vi "Speed PI Control.vi"() -> ()   [LabVIEW 2016]
uses:
  <vilib>/Platform/TimedLoop/XDataNode/timing_clust.ctl
  <vilib>/Platform/TimedLoop/XDataNode/nitl_modes.ctl
  <vilib>/Platform/TimedLoop/XDataNode/wakeup.ctl
  <vilib>/platform/TimedLoop/XDataNode/XDataNode.xnode
  <vilib>/Platform/TimedLoop/XDataNode/XDNodeRunTimeDep.lvlib
panel:
  in  "I-Gain":dbl(slide)=1.0 scale=0.0..2.0
  in  "P-Gain":dbl(slide)=1.0 scale=0.0..2.0
  in  "Setpoint Speed (rps)":dbl(slide) scale=-8.3..8.3
  out "Speed (rps)":dynamicdata(graph)
  in  "stop (F)":bool
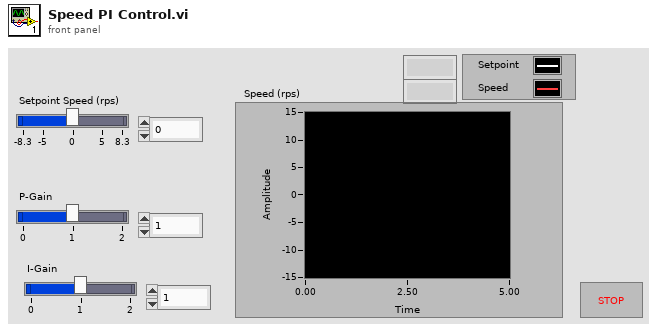
[diagram p1: front panel]
types:
  T1 = typedef "XDNodeRunTimeDep.lvlib/timing_clust.ctl" = cluster{"Expected End [f-1]":u64, "Actual End [f-1]":u64, "Finished Late? [f-1]":bool, "Expected End [i-1]":u64, "Actual End [i-1]":u64, "Finished Late? [i-1]":bool, "Expected Start [i]":u64, "Actual Start [i]":u64, "Expected Start [f]":u64, "Actual Start [f]":u64, "Source Name":string, "Structure Name":string, "Period":i64, "Deadline":i64, "Offset":i64, "Start":i64, "Priority":i32, "Timeout":i32, "Mode":T2, "Wakeup Reason":T3, "Error":errorcluster, "Source Type":string, "Secondary Source Type":string, "Global End Time":u64, "Global Start Time":u64, "Frame Duration":u64, "Iteration Duration":u64, "Assigned CPU":i32, "I/O Scan Engine Mode":u32}
  T2 = typedef "XDNodeRunTimeDep.lvlib/nitl_modes.ctl" = enum32{"No Change", "Process missed periods, maintain original phase", "Discard missed periods, maintain original phase", "Process missed periods, ignore original phase", "Discard missed periods, ignore original phase"}
  T3 = typedef "XDNodeRunTimeDep.lvlib/wakeup.ctl" = enum32{"Normal", "Aborted", "Asynchronous wakeup", "Timing source error", "Timed loop error", "Timeout"}
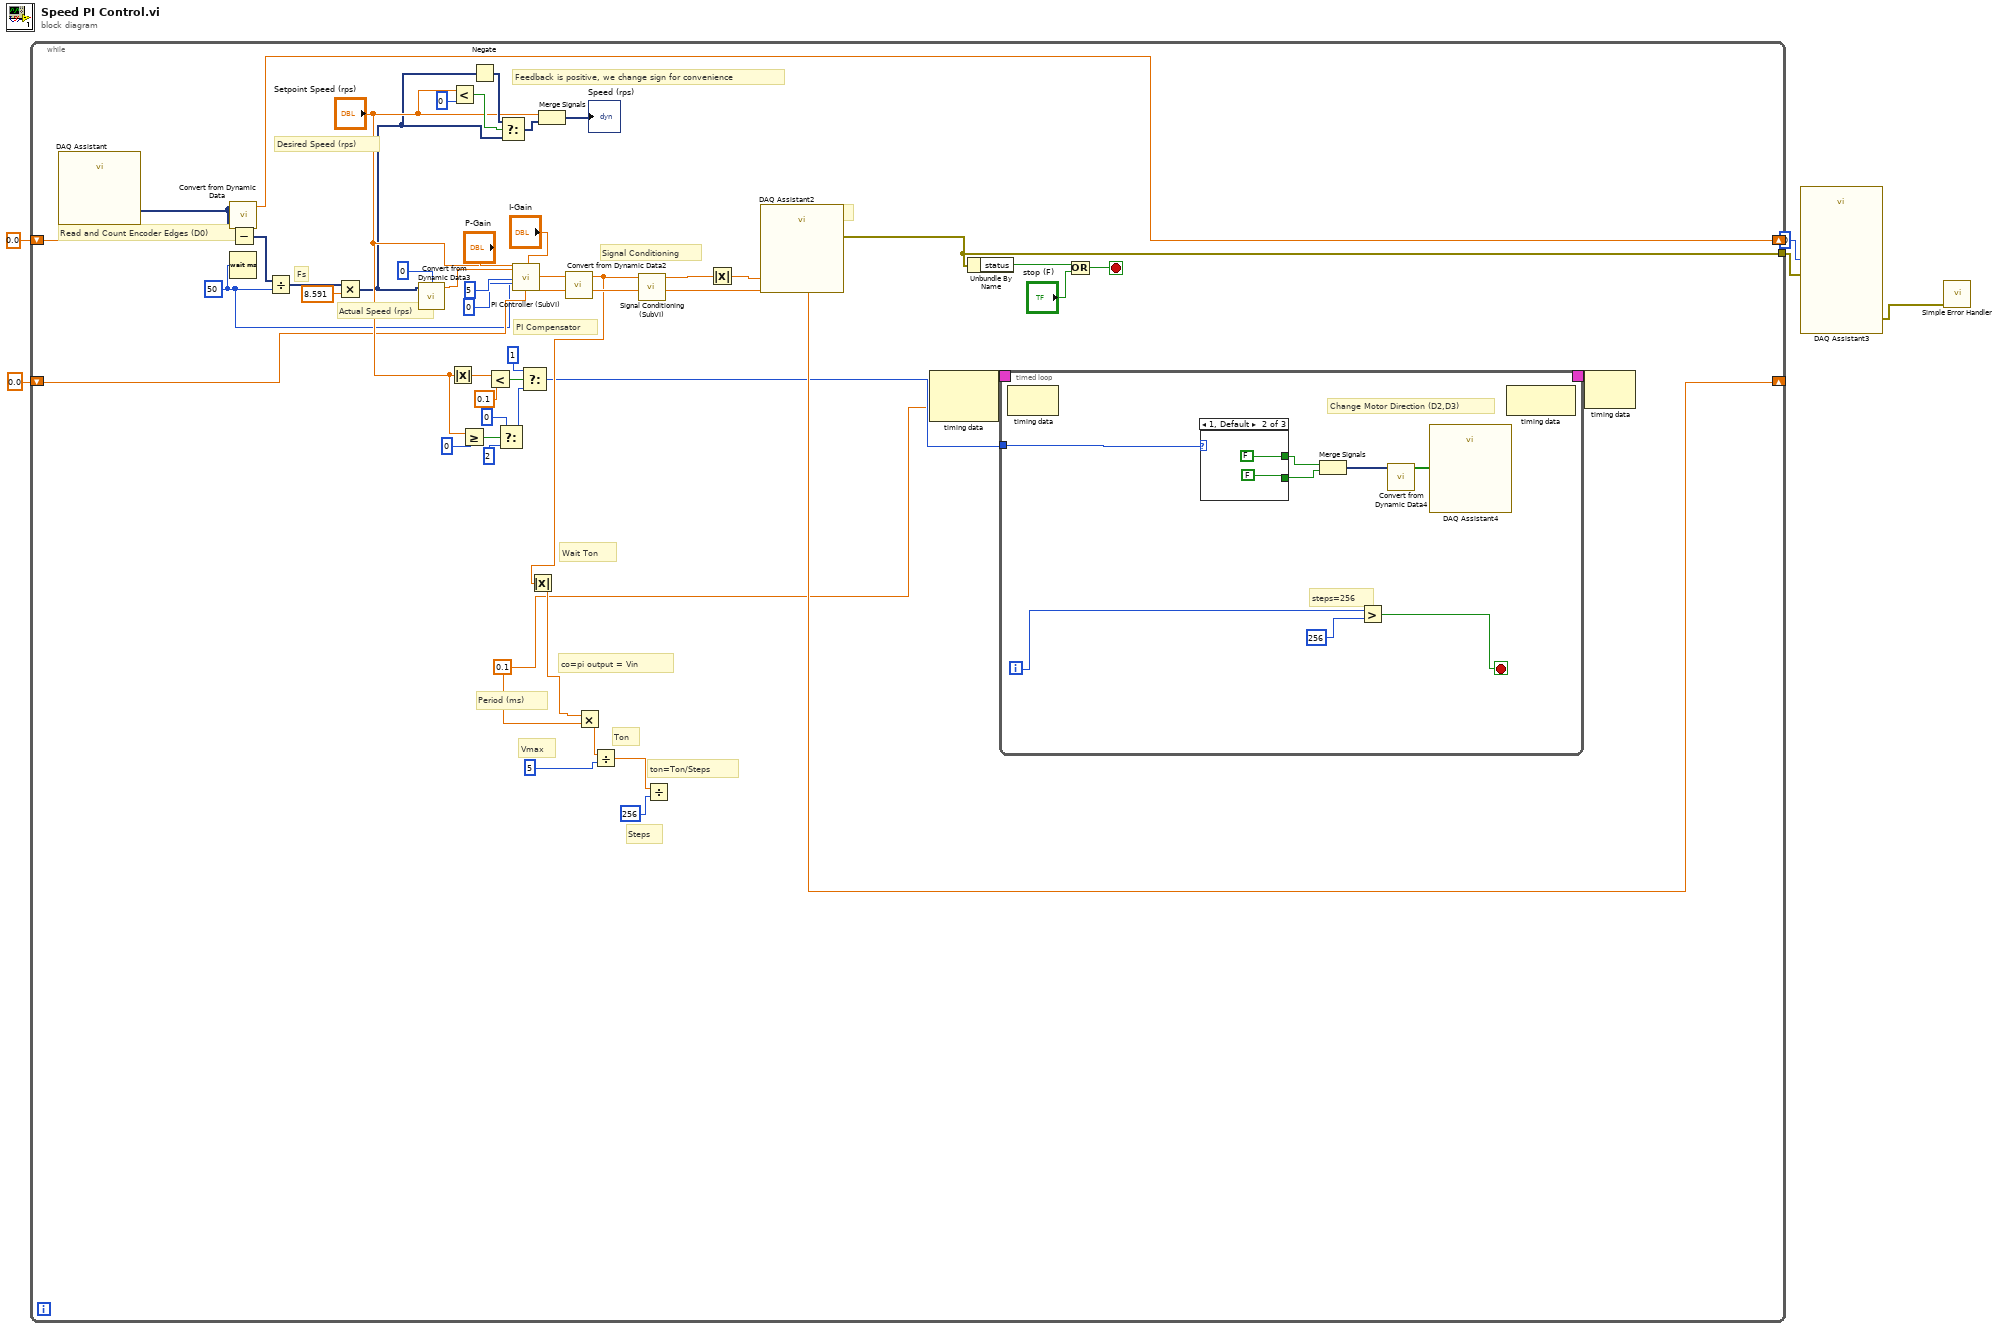
[diagram p0: block diagram]
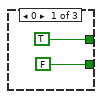
[diagram p2: hidden frame]
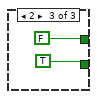
[diagram p3: hidden frame]
diagram:
  n1 = while {
    shift-right: [w53] -> _
    shift-left: 0.0 -> [w52]
    tunnel: [w48] -> w4
    shift-right: [w18] -> _
    shift-left: 0.0 -> [w21]
    stop <- w47 stop-if-true
    w6 = 0.1
    w20 = 50
    # "ton=Ton/Steps"
    # "Steps"
    # "Wait Ton"
    # "Ton"
    # "Vmax"
    # "co=pi output = Vin"
    # "Period (ms)"
    # "Desired Speed (rps)"
    # "Feedback is positive, we change sign for convenience"
    # "Signal Conditioning"
    # "PI Compensator"
    # "Fs"
    # "Actual Speed (rps)"
    # "Read and Count Encoder Edges (D0)"
    # "Plant Input (Ao0)"
    n2 = call "DAQ Assistant"() -> ("data"=w44:dynamicdata)  [unwired: 16 in, 3 out]
    n3 = call "Convert from Dynamic Data"("Dynamic Data Type"=w44) -> ("Scalar"=w53:dbl)  [unwired: 3 in]
    n4 = Wait (ms)(milliseconds to wait=w20) -> ()  [unwired: 1 out]
    n5 = Subtract(x=w44, y=w52) -> (x-y=w51:dynamicdata)
    n6 = Divide(x=w51, y=w20) -> (x/y=w50:dynamicdata)
    n7 = Multiply(x=w50, y=8.591) -> (x*y=w19:dynamicdata)
    n8 = call "Convert from Dynamic Data3"("Dynamic Data Type"=w19, "Channel"=0) -> ("Scalar"=w26:dbl)  [unwired: 2 in]
    n9 = Absolute Value(x="Setpoint Speed (rps)") -> (abs(x)=w38:dbl)
    n10 = Less?(x="Setpoint Speed (rps)", y=0) -> (x < y?=w29:bool)
    n11 = Greater Or Equal?(x="Setpoint Speed (rps)", y=0) -> (x >= y?=w41:bool)
    n12 = Negate(x=w19) -> (-x=w28:dynamicdata)
    n13 = Less?(x=w38, y=0.1) -> (x < y?=w36:bool)
    n14 = Select(t=0, s=w41, f=2) -> (s? t:f=w35:i32)
    n15 = Select(t=w28, s=w29, f=w19) -> (s? t:f=w30:dynamicdata)
    n16 = call "PI Controller (SubVI).vi"("sp"="Setpoint Speed (rps)", "pv"=w26, "maxim"=5, "minim"=0, "p"="P-Gain", "errsum"=w21, "i"="I-Gain", "h"=w20) -> ("output variable"=w17:dbl, "errsum"=w18:dbl)  [unwired: 18 in]
    n17 = Select(t=1, s=w36, f=w35) -> (s? t:f=w7:i32)
    n18 = Merge Signals("Setpoint Speed (rps)", w30) -> (→"Speed (rps)":dynamicdata)
    n19 = call "Convert from Dynamic Data2"("Dynamic Data Type"=w17) -> ("Scalar"=w13:dbl)  [unwired: 3 in]
    n20 = Absolute Value(x=w13) -> (abs(x)=w12:dbl)
    n21 = Multiply(x=w12, y=w6) -> (x*y=w16:dbl)
    n22 = Divide(x=w16, y=5) -> (x/y=w10:dbl)
    n23 = call "Signal Conditioning (SubVI).vi"("Input"=w13) -> ("Output"=w33:dbl)  [unwired: 10 in]
    n24 = Divide(x=w10, y=256) -> ()  [unwired: 1 out]
    n25 = Absolute Value(x=w33) -> (abs(x)=w34:dbl)
    n26 = call "DAQ Assistant2"("data"=w34) -> ("error out"=w48:errorcluster)  [unwired: 17 in, 1 out]
    n27 = node-c288(w6) -> (w9:T1)  [unwired: 1 in]
    n28 = Unbundle By Name(w48) -> ("status"=w45:bool)
    n29 = timed-loop {
      timing: w9 -> [_]
      timing-out: [_] -> w8
      tunnel: w7 -> [w57]
      i -> [w56]
      stop <- w54 stop-if-true
      # "steps=256"
      # "Change Motor Direction (D2,D3)"
      n30 = node-c288() -> ()  [unwired: 1 in, 1 out]
      n31 = case shown="1, Default" w57 {
        tunnel: [TRUE FALSE FALSE] -> w59
        tunnel: [FALSE FALSE TRUE] -> w58
        frame 0 {
        }
        frame 1, Default {
        }
        frame 2 {
        }
      }
      n32 = Merge Signals(w59, w58) -> (w61:dynamicdata)
      n33 = Greater?(x=w56, y=256) -> (0:w54:bool)
      n34 = call "Convert from Dynamic Data4"("Dynamic Data Type"=w61) -> ("Array"=w60:bool[])  [unwired: 3 in]
      n35 = call "DAQ Assistant4"("data"=w60) -> ()  [unwired: 17 in, 2 out]
      n36 = node-c288() -> ()  [unwired: 1 in, 1 out]
    }
    n37 = Or(x=w45, y="stop (F)") -> (x .or. y?=w47:bool)
    n38 = node-c288(w8) -> ()  [unwired: 1 out]
  }
  n39 = call "DAQ Assistant3"("data"=0, "error in"=w4) -> ("error out"=w2:errorcluster)  [unwired: 16 in, 1 out]
  n40 = call <vilib>:"Simple Error Handler.vi"("error in (no error)"=w2) -> ()  [unwired: 4 in, 5 out]
